vi "FTW-Producer-Construct.vi"(5 "Server Address":string, 7 "Identity":string, 11 "error in":errorcluster) -> (4 "FTW-Producer Out":refnum<class "FTW-Producer.lvclass">, 15 "error out":errorcluster)   [LabVIEW 2013, in "FTW-Producer.lvclass"]
uses:
  FTW-Producer.lvclass
  Ether/FTW-Ether-EndpointType.ctl
  Endpoint/FTW-Endpoint.lvclass
  FTW-Producer.lvclass/FTW-Producer.ctl
  Ether/FTW-Ether.lvclass
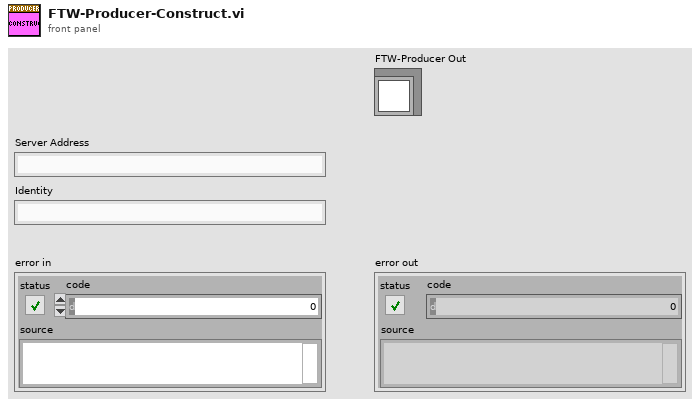
[diagram p1: front panel]
types:
  T1 = typedef "FTW-Ether.lvclass/FTW-Ether-EndpointType.ctl" = enum16{"Server", "Client", "Publisher", "Subscriber"}
  T2 = typedef "FTW-Ether.lvclass/FTW-Ether-MessageTransportScheme.ctl" = enum16{"LabVIEW Queues (lvq://)", "TCP (tcp://)"}
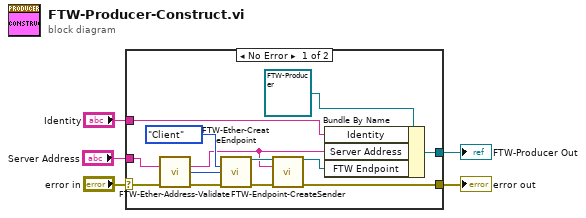
[diagram p0: block diagram]
diagram:
  n1 = case shown="No Error" "error in" {
    selector: "error in" -> [w16 w19]
    tunnel: [w9 w19] -> w3
    tunnel: [w17 _] -> w5
    tunnel: "Server Address" -> [w12 _]
    tunnel: "Identity" -> [w10 _]
    frame No Error {
      n2 = call "FTW-Ether-Address-Validate.vi"("Address"=w12, "error in"=w16) -> ("Sanitized Address"=w6:string, "Message Transport Scheme"=w13:T2, "error out"=w15:errorcluster)  [unwired: 11 in]
      n3 = call "FTW-Ether-CreateEndpoint.vi"("Endpoint Type"=FTW-Ether-EndpointType."Client", "Message Transport Scheme"=w13, "error in"=w15) -> ("FTW Endpoint"=w8:refnum<class "FTW-Endpoint.lvclass">, "error out"=w11:errorcluster)  [unwired: 11 in]
      n4 = call-dynamic "FTW-Endpoint-CreateSender.vi"("FTW Endpoint"=w8, "Endpoint Address"=w6, "error in"=w11) -> ("FTW Endpoint out"=w7:refnum<class "FTW-Endpoint.lvclass">, "error out"=w9:errorcluster)  [unwired: 11 in]
      n5 = Bundle By Name(cluster=refnum<class "FTW-Producer.lvclass"> refnum ("LVmsg_Client in"), "Identity"=w10, "Server Address"=w6, "FTW Endpoint"=w7) -> (w17:refnum<class "FTW-Producer.lvclass">)
    }
    frame Error {
    }
  }
  "FTW-Producer Out" <- w5
  "error out" <- w3
